vi "Default Value State Name.vi"() -> (4 "set default value state":string, 6 "initialize state":string, 8 "post ui update":string, 10 "load values":string)   [LabVIEW 2021, in "Converter Reusables.lvlib"]
uses:
  Converter Reusables.lvlib
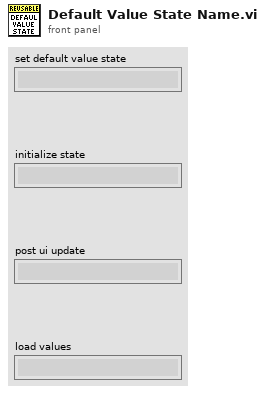
[diagram p1: front panel]
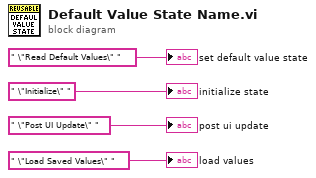
[diagram p0: block diagram]
diagram:
  "set default value state" <- " \"Read Default Values\" " ("element")
  "initialize state" <- " \"Initialize\" " ("new element/subarray")
  "post ui update" <- " \"Post UI Update\" " ("new element/subarray")
  "load values" <- " \"Load Saved Values\" " ("new element/subarray")
